vi "Stop Button Scroll.vi"(8 "error in (no error)":errorcluster, 11 "SwipeMenu in":refnum<class "SwipeMenu.lvclass">) -> (0 "error out":errorcluster, 3 "SwipeMenu out":refnum<class "SwipeMenu.lvclass">)   [LabVIEW 2019, in "SwipeMenu.lvclass"]
uses:
  SwipeMenu.lvclass
  SwipeMenu.lvclass/SwipeMenu.ctl
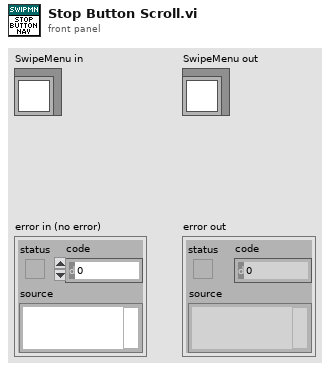
[diagram p1: front panel]
types:
  T1 = enum16{"Idle", "Mouse Nav", "Slowdown", "Button Nav"}
  T2 = typedef "SwipeMenu.lvclass/State Data.ctl" = cluster{"State":enum16{"Idle", "Mouse Nav", "Slowdown", "Button Nav"}, "Timeout":i32, "Time":timestamp, "Position":i32, "Scroll Position":i16, "Rate":dbl, "Direction":enum16{"Left", "Right"}}
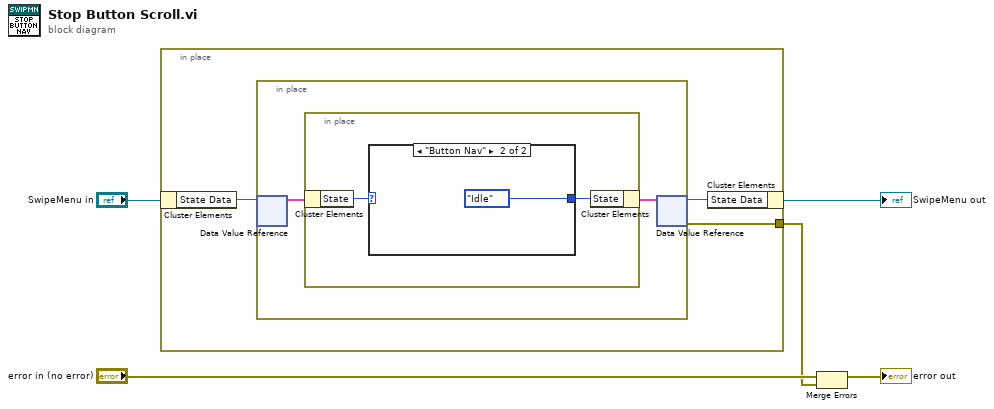
[diagram p0: block diagram]
diagram:
  n1 = in-place {
    in-place-border: [w6] -> w1
    n2 = in-place-cluster #1("SwipeMenu in") -> ("State Data"=w8:refnum<data-value>)
    n3 = in-place {
      n4 = in-place-dvr #2(w8) -> (w10:T2)  [unwired: 1 out]
      n5 = in-place {
        n6 = in-place-cluster #3(w10) -> ("State"=w12:T1)
        n7 = case shown="\"Button Nav\"" w12 {
          selector: w12 -> [w13 _]
          tunnel: [w13 T1."Idle" ("State")] -> w11
          frame Default {
          }
          frame "Button Nav" {
          }
        }
        n8 = in-place-cluster #3("State"=w11) -> (w9:T2)
      }
      n9 = in-place-dvr #2(w9) -> (w7:refnum<data-value>, w6:errorcluster)
    }
    n10 = in-place-cluster #1("State Data"=w7) -> (→"SwipeMenu out":refnum<class "SwipeMenu.lvclass">)
  }
  n11 = Merge Errors("error in (no error)", w1) -> (→"error out":errorcluster)
